vi "read_waveform_number.vi"(1 "path":string) -> (0 "length":i32)   [LabVIEW 2022 SP3]
uses:
  <vilib>/Waveform/WDTFileIO.llb/Read Waveform from File.vi
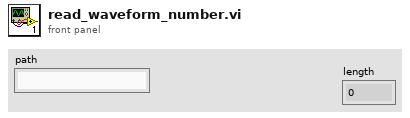
[diagram p1: front panel]
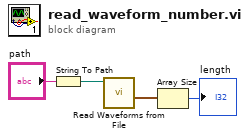
[diagram p0: block diagram]
diagram:
  n1 = String To Path(string="path") -> (path=w4:path)
  n2 = call-poly <vilib>:"Read Waveforms from File.vi"("file path (dialog if empty)"=w4) -> ("all waveforms in record"=w1:waveform(dbl)[])  [unwired: 5 in, 3 out]
  n3 = Array Size(array=w1) -> (size(s)=→"length":i32)
